vi "仁莫密封检测系统.vi"() -> ()   [LabVIEW 2020]
uses:
  <vilib>/event_ctls.llb/eventvkey.ctl
  <vilib>/NI/Modbus Library/API/Master/Modbus Master.lvclass
  <vilib>/Utility/file.llb/Read Delimited Spreadsheet (string).vi
  <vilib>/NI/Modbus Library/Transmission Data Unit/RTU/RTU Data Unit.lvclass
  <vilib>/NI/Modbus Library/Master Function Definition/Master Function Definition.lvclass
  <vilib>/NI/Modbus Library/Network Protocol/Network Master/Serial/Serial Master.lvclass
panel:
  in  "扫码数据":string
  out "MES状态":bool
  out "通讯状态":bool
  out "刷新按钮":bool
  out "参数组别":string
  out "测试时间":string
  out "实时压力":string
  out "泄露压力":string
  out "门限压力":string
  out "目标压力":string
  out "测试 NG":string
  out "测试 OK":string
  out "测试结果":string
  out "测试总量":string
  out "实时压力(图)":dbl(graph)
  in  "清除计数":bool
  in  "设备启动":bool
  out "消息框":string
  in  "设备停止":bool
  in  "阻断通讯":bool=TRUE
  out "运行状态":string
  out "失败原因":string
  in  "Exit":bool
  # "仁 莫 密 封 检 测 系 统"
  # "S"
  # "Pa"
  # "Pa"
  # "Pa"
  # "Pa"
  # "pcs"
  # "pcs"
  # "pcs"
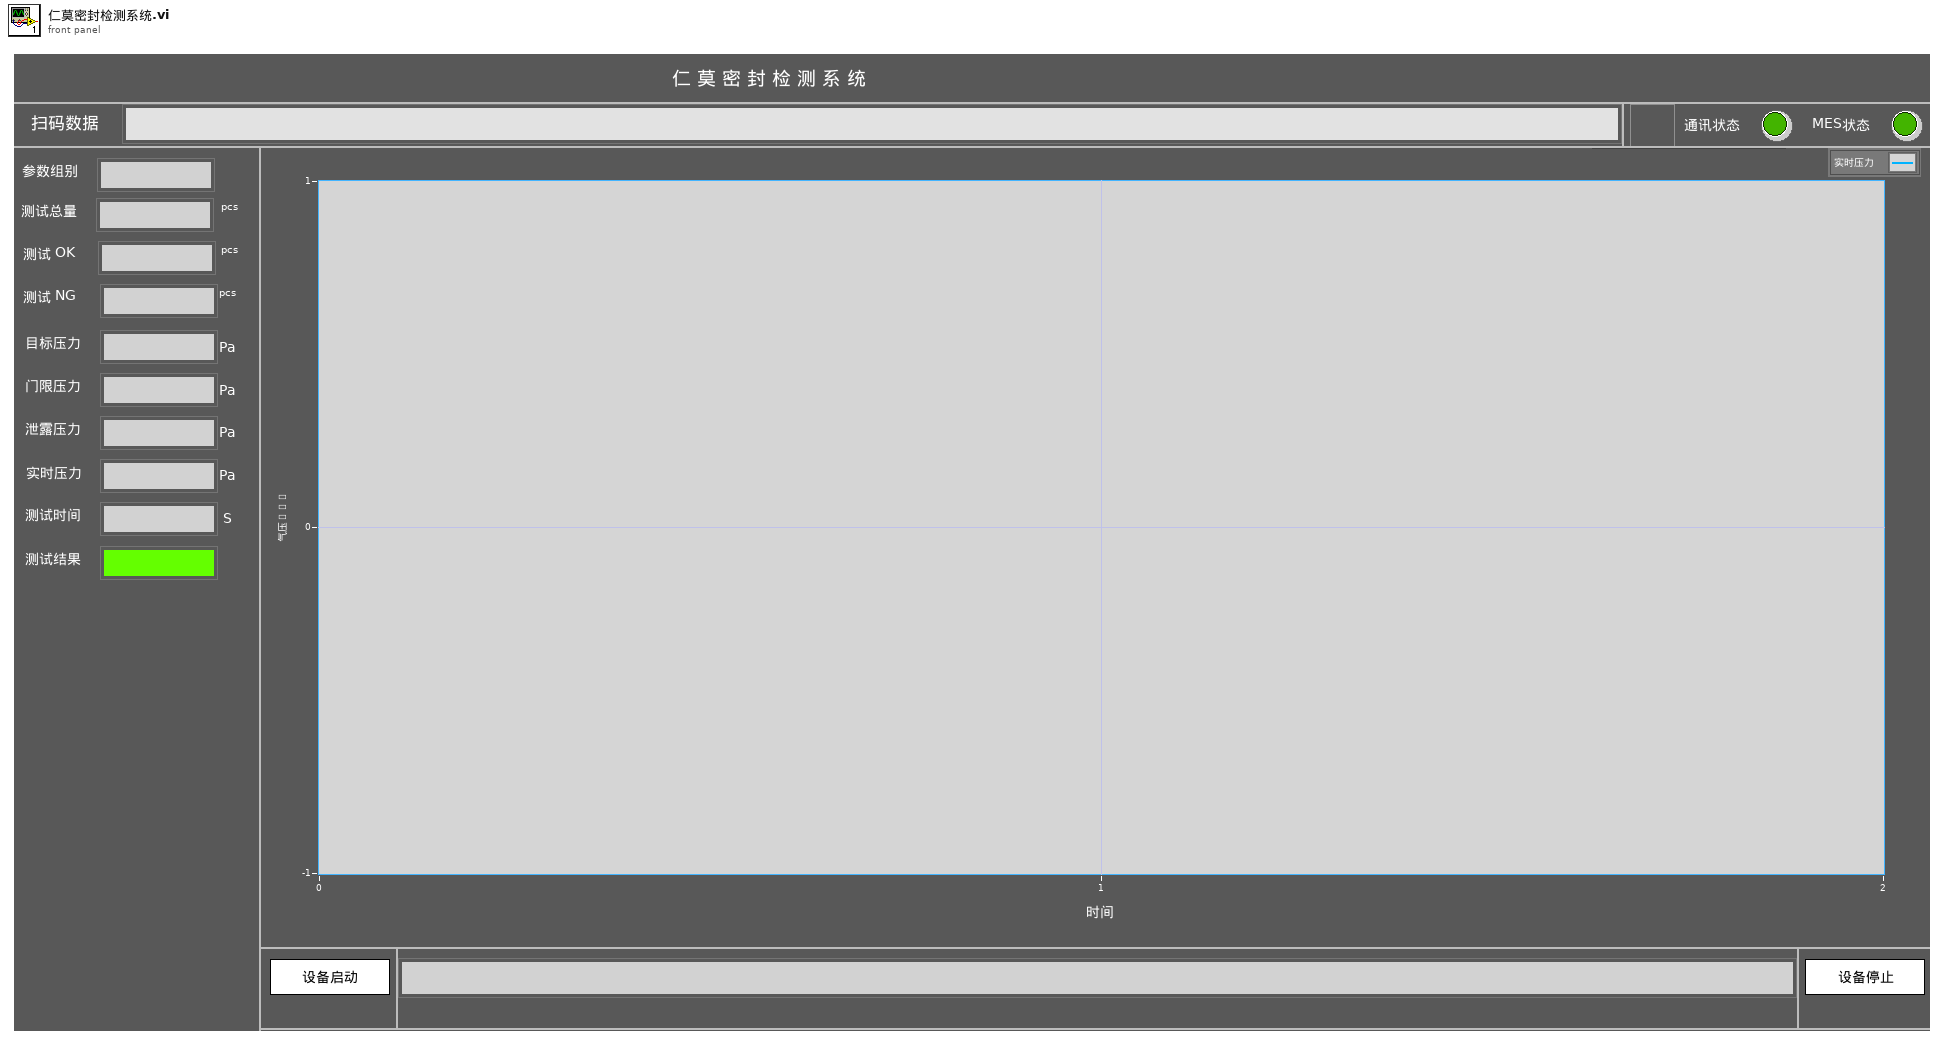
[diagram p1: front panel]
types:
  T1 = typedef "eventvkey.ctl" = enum16{"ASCII", "Enter", "Return", "Shift", "Ctrl", "Alt", "Cmd", "Opt", "Caps", "NumLock", "Clear", "Break", "Up", "Down", "Left", "Right", "Insert", "Delete", "Home", "End", "PageUp", "PageDown", "Escape", "Help", "Pause", "ScrollLock", "F1", "F2", "F3", "F4", "F5", "F6", "F7", "F8", "F9", "F10", "F11", "F12", "F13", "F14", "F15", "F16", "F17", "F18", "F19", "F20", "F21", "F22", "F23", "F24", "Play", "VolumeUp", "VolumeDown", "Mute", "Two Byte Char"}
  T2 = cluster{"地址":u16, "数量":u16, "寄存器值":u16[], "产品总数":string}[]
  T3 = enum32{"Invalid", "Standard", "Closed", "Hidden", "Minimized", "Maximized"}
  T4 = enum32{"invalid app kind", "Development System", "Run Time System", "Student Edition", "Embedded LabVIEW", "Evaluation", "Custom"}
  T5 = cluster{"地址":u16, "数量":u16, "寄存器值":u16[], "名称":string}[]
  T6 = cluster{"读取信息簇":cluster{"地址":u16, "数量":u16, "寄存器值":u16[], "名称":string}, "值解析":string}[]
  T7 = cluster{"温度instance":refnum<class "Modbus Master.lvclass">, "Core":cluster{"Current VI Reference":refnum<vi>, "Close Panel on Exit?":bool}, "serial master instance":refnum<class "Modbus Master.lvclass">, "进站OK":bool, "连接成功":bool, "正在运行":bool, "用户登录":bool, "A读保持寄存器信息组":cluster{"地址":u16, "数量":u16, "寄存器值":u16[], "名称":string}[], "A写入线圈信息组":cluster{"地址":u16, "布尔":bool, "名称":string}[], "A读多组线圈信息组":cluster{"地址":u16, "数量":u16, "名称":string, "线圈组":bool[]}[]}
  T8 = cluster{"连接成功":bool, "MB_实体":refnum<class "Modbus Master.lvclass">}
  T9 = cluster{"地址":u16, "数量":u16, "名称":string, "线圈组":bool[]}[]
  T10 = cluster{"Current VI Reference":refnum<vi>, "Close Panel on Exit?":bool}
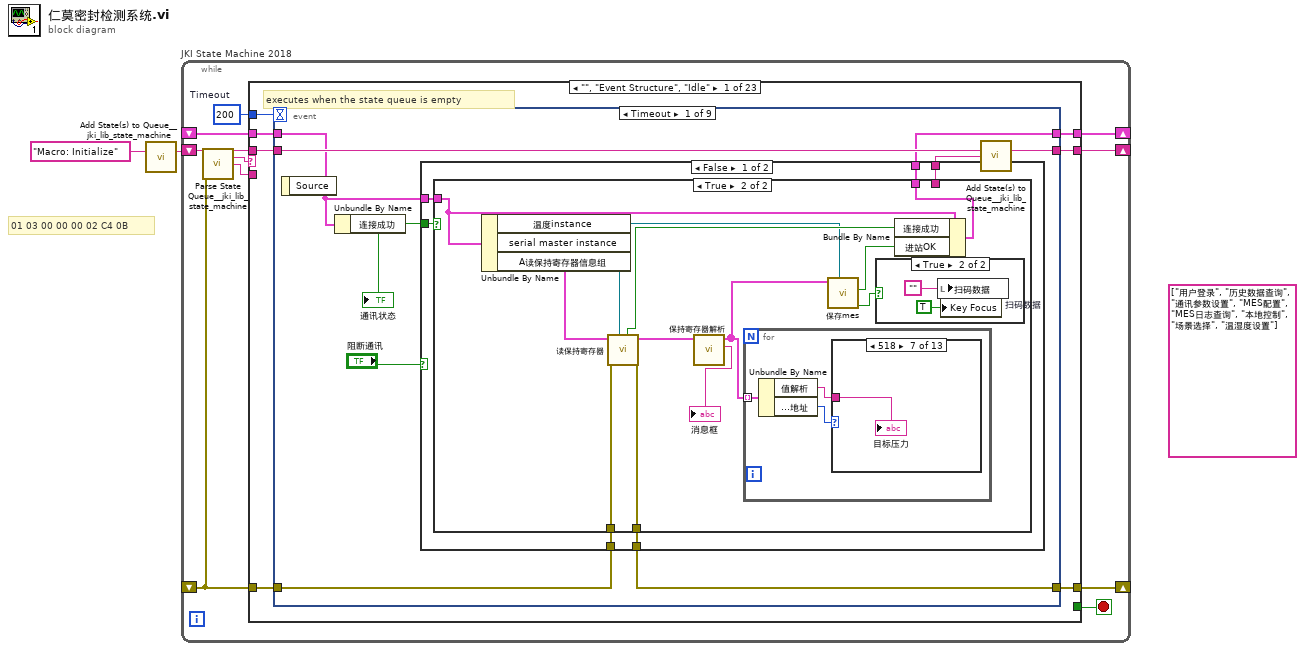
[diagram p0: block diagram]
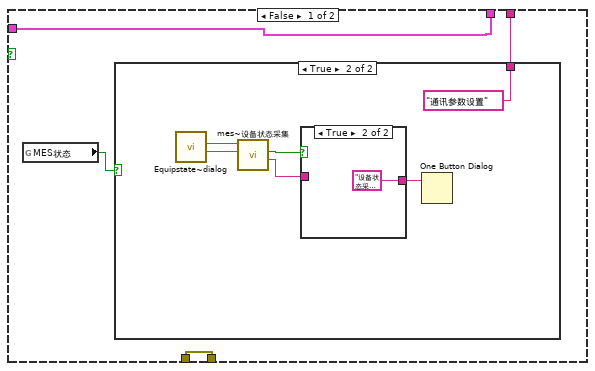
[diagram p2: hidden frame]
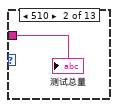
[diagram p7: hidden frame]
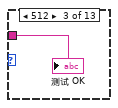
[diagram p8: hidden frame]
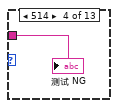
[diagram p9: hidden frame]
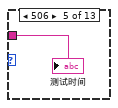
[diagram p10: hidden frame]
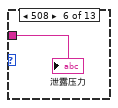
[diagram p11: hidden frame]
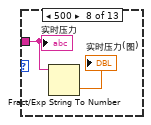
[diagram p12: hidden frame]
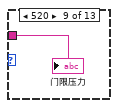
[diagram p13: hidden frame]
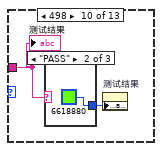
[diagram p14: hidden frame]
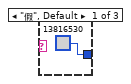
[diagram p15: hidden frame]
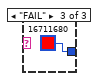
[diagram p16: hidden frame]
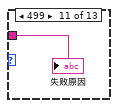
[diagram p17: hidden frame]
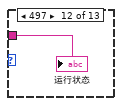
[diagram p18: hidden frame]
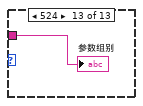
[diagram p19: hidden frame]
diagram:
  (unwired) string[] ["用户登录", "历史数据查询", "通讯参数设置", "MES配置", "MES日志查询", "本地控制", "场景选择", "温湿度设置"] ("L10n_item tags 1")
  # "01 03 00 00 00 02 C4 0B"
  n1 = call <vilib>:"Add State(s) to Queue__jki_lib_state_machine.vi"("State(s) in (\"\")"="Macro: Initialize") -> ("States Out"=w2:string)  [unwired: 14 in]
  n2 = while "JKI State Machine 2018" {
    shift-right: [w6] -> _
    shift-left: _ -> [w5]
    shift-right: [w9] -> _
    shift-left: _ -> [w3]
    shift-right: [w8] -> _
    shift-left: w2 -> [w10]
    stop <- w7 stop-if-true
    w4 = 200  # Timeout
    n3 = call <vilib>:"Parse State Queue__jki_lib_state_machine.vi"("State Queue"=w10, "Error In (no error)"=w3) -> ("Remaining States"=w12:string, "Current State"=w13:string, "Arguments"=w11:string)  [unwired: 11 in]
    n4 = case shown="\"\", \"Event Structure\", \"Idle\"" w13 {
      selector: w13 -> [_ _ w224 _ _ _ _ _ _ _ _ _ _ _ _ _ _ _ _ _ _ _ _]
      tunnel: w12 -> [w20 w223 w228 w247 w254 w259 w263 w284 w292 w296 w310 w316 w327 w396 w401 w411 w416 w432 w458 w507 w550 w562 w567]
      tunnel: w11 -> [_ _ _ _ _ _ _ _ _ _ _ w311 w321 _ _ _ _ _ _ _ _ _ _]
      tunnel: w5 -> [w18 w220 w226 w240 w251 w257 w260 _ w288 w293 w308 w314 w323 w393 w398 w408 w413 w426 w452 w501 w543 w559 w564]
      tunnel: [w17 w221 w230 w244 errorcluster {"status"=FALSE, "code"=0, "source"=""} ("error out") w256 w261 w281 w289 w294 w307 w312 w324 w394 w399 w409 w414 w422 w455 w504 w547 w560 w565] -> w9
      tunnel: w3 -> [w16 w221 w229 w244 w249 w256 w261 w281 w286 w294 w307 w313 w325 w394 w399 w409 w414 w429 w456 w505 w548 w560 w565]
      tunnel: [w19 w222 w227 w246 w253 w258 w262 w283 w291 w295 w309 w315 w326 w395 w400 w410 w415 w431 w457 w506 w549 w561 w566] -> w8
      tunnel: [_ _ _ _ _ TRUE _ _ _ _ _ _ _ _ _ _ _ _ _ _ _ _ _] -> w7
      tunnel: [w15 w220 w226 w245 w251 w257 w260 w282 w288 w293 w308 w314 w323 w393 w398 w408 w413 w424 w450 w499 w544 w559 w563] -> w6
      tunnel: w4 -> [w14 _ _ _ _ _ _ _ _ _ _ _ _ _ _ _ _ _ _ _ _ _ _]
      frame "", "Event Structure", "Idle" {
        # "executes when the state queue is empty"
        n5 = event shown="[0] Timeout" {
          selector: _ -> [_ _ _ _ _ _ _ _ _]
          dyn-events: _ -> [_ _ _ _ _ _ _ _ _]
          timeout: w14 -> [_ _ _ _ _ _ _ _ _]
          tunnel: w20 -> [w29 w89 w94 w100 w181 w193 w203 w213 w219]
          tunnel: [w28 w88 w93 w99 w180 w194 w202 w212 w218] -> w19
          tunnel: w18 -> [w27 w86 w91 w96 w177 w192 w198 w210 w216]
          tunnel: [w25 w87 w92 w98 w179 w191 w195 w211 w217] -> w17
          tunnel: w16 -> [w26 w87 w92 w98 w179 w191 w196 w211 w217]
          tunnel: [w24 w86 w91 w95 w176 w192 w197 w210 w216] -> w15
          event Timeout {
            n6 = event-data() -> ()  [unwired: 1 in, 1 out]
            n7 = Unbundle By Name(w27) -> ("连接成功"=w22:bool)
            "通讯状态" <- w22
            n8 = case shown="False" "阻断通讯" {
              tunnel: w22 -> [w35 _]
              tunnel: w27 -> [w34 w83]
              tunnel: w26 -> [w33 w84]
              tunnel: [w32 w84] -> w25
              tunnel: [w31 w83] -> w24
              tunnel: [w30 _] -> w21
              frame False {
                n9 = case shown="True" w35 {
                  tunnel: w34 -> [w37 w58]
                  tunnel: w33 -> [w39 w60]
                  tunnel: [w39 w59] -> w32
                  tunnel: [w37 w52] -> w31
                  tunnel: [w36 _] -> w30
                  frame False {
                    n10 = global read "Global.vi" "MES状态"() -> (w38:bool)
                    n11 = case shown="True" w38 {
                      tunnel: [_ "通讯参数设置"] -> w36
                      frame False {
                      }
                      frame True {
                        n12 = call "Equipstate~dialog.vi"() -> ("RecordDate"=w44:string, "Equipstate"=w45:string)  [unwired: 10 in]
                        n13 = call "mes~设备状态采集.vi"("RecordDate"=w44, "设备状态"=w45) -> ("ErrorMessage"=w42:string, "设备状态采集成功"=w43:bool)  [unwired: 7 in, 1 out]
                        n14 = case shown="True" w43 {
                          tunnel: w42 -> [w46 _]
                          tunnel: [w46 "设备状态采集成功。"] -> w41
                          frame False {
                          }
                          frame True {
                          }
                        }
                        n15 = One Button Dialog(message=w41) -> ()  [unwired: 1 in, 1 out]
                      }
                    }
                  }
                  frame True {
                    n16 = Unbundle By Name(w58) -> ("温度instance"=w49:refnum<class "Modbus Master.lvclass">, "serial master instance"=w57:refnum<class "Modbus Master.lvclass">, "A读保持寄存器信息组"=w56:T5)
                    n17 = call "读保持寄存器.vi"("MB_实体"=w57, "error in"=w60, "读保持寄存器信息组__输入"=w56) -> ("输出簇"=w59:errorcluster, "读保持寄存器信息组_输出"=w54:T5, "连接成功"=w55:bool)  [unwired: 6 in]
                    n18 = call "保持寄存器解析.vi"("A读保持寄存器信息组"=w54) -> ("运行状态"=→"消息框":string, "参数值"=w51:T6)  [unwired: 9 in]
                    n19 = for {
                      tunnel: w51 -> [w64] mode=indexing
                      n20 = Unbundle By Name(w64) -> ("值解析"=w63:string, "读取信息簇.地址"=w65:u16)
                      n21 = case shown="518" w65 {
                        tunnel: w63 -> [_ w66 w67 w68 w69 w70 w71 w73 w74 w76 w80 w81 w82]
                        frame Default {
                        }
                        frame 510 {
                          "测试总量" <- w66
                        }
                        frame 512 {
                          "测试 OK" <- w67
                        }
                        frame 514 {
                          "测试 NG" <- w68
                        }
                        frame 506 {
                          "测试时间" <- w69
                        }
                        frame 508 {
                          "泄露压力" <- w70
                        }
                        frame 518 {
                          "目标压力" <- w71
                        }
                        frame 500 {
                          n22 = Fract/Exp String To Number(string=w73) -> (number=→"实时压力(图)":dbl)  [unwired: 3 in, 1 out]
                          "实时压力" <- w73
                        }
                        frame 520 {
                          "门限压力" <- w74
                        }
                        frame 498 {
                          n23 = case shown="\"PASS\"" w76 {
                            tunnel: [u32 13816530 ("颜色盒") u32 6618880 u32 16711680] -> w75
                            frame "假", Default {
                            }
                            frame "PASS" {
                            }
                            frame "FAIL" {
                            }
                          }
                          n24 = property on="测试结果" class="Str"("Text.BGColor"=w75) -> ()  [unwired: 2 in, 2 out]
                          "测试结果" <- w76
                        }
                        frame 499 {
                          "失败原因" <- w80
                        }
                        frame 497 {
                          "运行状态" <- w81
                        }
                        frame 524 {
                          "参数组别" <- w82
                        }
                      }
                    }
                    n25 = call "保存mes.vi"("温度instance"=w49, "参数值"=w51) -> ("已保存?"=w48:bool, "进站OK?"=w50:bool)  [unwired: 8 in]
                    n26 = case shown="True" w48 {
                      frame False {
                      }
                      frame True {
                        n27 = local write "扫码数据"("") -> ()
                        n28 = property on="扫码数据" class="Str"("Key Focus"=TRUE) -> ()  [unwired: 2 in, 2 out]
                      }
                    }
                    n29 = Bundle By Name(cluster=w58, "连接成功"=w55, "进站OK"=w50) -> (w52:T7)
                  }
                }
              }
              frame True {
              }
            }
            n30 = call <vilib>:"Add State(s) to Queue__jki_lib_state_machine.vi"("State(s) in (\"\")"=w29, "State(s) at Back (\"\")"=w21) -> ("States Out"=w28:string)  [unwired: 13 in]
          }
          event "设备启动": Value Change {
            n31 = event-data() -> ()  [unwired: 1 in, 1 out]
            n32 = call <vilib>:"Add State(s) to Queue__jki_lib_state_machine.vi"("State(s) in Front (\"\")"="//Communication: 读运行标志\nCommunication: 设备启动\n//Communication: 读运行标志", "State(s) in (\"\")"=w89) -> ("States Out"=w88:string)  [unwired: 13 in]
          }
          event "设备停止": Value Change {
            n33 = event-data() -> ()  [unwired: 1 in, 1 out]
            n34 = call <vilib>:"Add State(s) to Queue__jki_lib_state_machine.vi"("State(s) in Front (\"\")"="//Communication: 读运行标志\nCommunication: 设备停止\n//Communication: 读运行标志", "State(s) in (\"\")"=w94) -> ("States Out"=w93:string)  [unwired: 13 in]
          }
          event Menu Selection (User) {
            n35 = event-data() -> ("ItemTag"=w97:string)  [unwired: 1 in]
            n36 = case shown="\"本地控制\"" w97 {
              tunnel: w96 -> [w101 w104 w112 w123 w135 w137 w148 w161 w166]
              tunnel: [w101 w103 w112 w123 w135 w136 w147 w161 w165] -> w95
              frame "假", Default {
              }
              frame "用户登录" {
                n37 = call "mes~Login Dialog.vi"() -> ("Success?"=w102:bool)  [unwired: 10 in, 1 out]
                n38 = Bundle By Name(cluster=w104, "用户登录"=w102) -> (w103:T7)
                n39 = case shown="True" w102 {
                  frame False {
                    n40 = Current VI's Menubar() -> (w106:refnum<k9>)
                    n41 = Delete Menu Items(9:w106) -> (3:w105:refnum<k9>)  [unwired: 3 in, 1 out]
                    n42 = Insert Menu Items(7:string[] ["用户登录", "历史数据查询", "MES配置", "MES日志查询", "本地控制", "温湿度设置"] ("L10n_item tags 1"), 9:w105) -> ()  [unwired: 4 in, 3 out]
                  }
                  frame True {
                    n43 = Current VI's Menubar() -> (w110:refnum<k9>)
                    n44 = Delete Menu Items(9:w110) -> (0:w108:errorcluster, 3:w109:refnum<k9>)  [unwired: 3 in]
                    n45 = Insert Menu Items(6:w108, 7:string[] ["用户登录", "历史数据查询", "通讯参数设置", "MES配置", "MES日志查询", "本地控制"] ("L10n_item tags 1"), 9:w109) -> ()  [unwired: 3 in, 3 out]
                  }
                }
              }
              frame "历史数据查询" {
                n46 = stacked-sequence {
                  frame #0 {
                    n47 = call <vilib>:"Check if File or Folder Exists.vi"("path"=path "D:/MES" ("路径")) -> ("file or folder exists?"=w115:bool, "dup path"=w114:path)  [unwired: 8 in, 1 out]
                    n48 = case shown="False" w115 {
                      tunnel: w114 -> [w117 w118]
                      tunnel: [w116 w118] -> _
                      frame False {
                        n49 = Create Folder(path (use dialog)=w117) -> (created path=w116:path)  [unwired: 2 in, 2 out]
                      }
                      frame True {
                      }
                    }
                  }
                  frame #1 {
                    n50 = call <vilib>:"Space Constant.vi"() -> ("String"=w120:string)
                    n51 = Concatenate Strings("explorer" ("字符串"), w120, "D:\\MES" ("字符串")) -> (w122:string)
                    n52 = call <vilib>:"System Exec.vi"("command line"=w122) -> ()  [unwired: 7 in, 4 out]
                  }
                }
              }
              frame "MES日志查询" {
                n53 = stacked-sequence {
                  frame #0 {
                    n54 = call <vilib>:"Check if File or Folder Exists.vi"("path"=path "D:/Log" ("路径")) -> ("file or folder exists?"=w126:bool, "dup path"=w125:path)  [unwired: 8 in, 1 out]
                    n55 = case shown="False" w126 {
                      tunnel: w125 -> [w128 w129]
                      tunnel: [w127 w129] -> _
                      frame False {
                        n56 = Create Folder(path (use dialog)=w128) -> (created path=w127:path)  [unwired: 2 in, 2 out]
                      }
                      frame True {
                      }
                    }
                  }
                  frame #1 {
                    n57 = call <vilib>:"Space Constant.vi"() -> ("String"=w131:string)
                    n58 = Concatenate Strings("explorer" ("字符串"), w131, "D:\\Log" ("字符串")) -> (w133:string)
                    n59 = call <vilib>:"System Exec.vi"("command line"=w133) -> ()  [unwired: 7 in, 4 out]
                  }
                }
              }
              frame "MES配置" {
                n60 = call "mes配置前验证.vi"() -> ("Success?"=w134:bool)  [unwired: 10 in, 1 out]
                n61 = case shown="True" w134 {
                  frame False {
                  }
                  frame True {
                    n62 = call "mes参数配置.vi"() -> ()  [unwired: 11 in, 1 out]
                  }
                }
              }
              frame "通讯参数设置" {
                n63 = stacked-sequence {
                  tunnel: w137 -> [_ w142 _]
                  tunnel: [_ w139 _] -> w136
                  frame #0 {
                    n64 = local write "阻断通讯"(TRUE ("阻断通讯")) -> ()
                  }
                  frame #1 {
                    n65 = call "通讯参数设置.vi"() -> ("A设备簇"=w143:T8)  [unwired: 5 in]
                    n66 = Unbundle By Name(w143) -> ("MB_实体"=w141:refnum<class "Modbus Master.lvclass">, "连接成功"=w140:bool)
                    n67 = Bundle By Name(cluster=w142, "serial master instance"=w141, "连接成功"=w140) -> (w139:T7)
                  }
                  frame #2 {
                    n68 = local write "阻断通讯"(FALSE ("阻断通讯")) -> ()
                  }
                }
              }
              frame "本地控制" {
                n69 = call "本地控制.vi"() -> ("远程2"=w146:bool)  [unwired: 11 in]
                "MES状态" <- w146
                n70 = Not(x=w146) -> (.not. x?=w145:bool)
                n71 = Bundle By Name(cluster=w148, "用户登录"=w145, "进站OK"=w145) -> (w147:T7)
                n72 = global write "Global.vi" "MES状态"(w146) -> ()
                n73 = global write "Global.vi" "产品进站"(w145) -> ()
                n74 = case shown="True" w146 {
                  frame False {
                    n75 = Current VI's Menubar() -> (w150:refnum<k9>)
                    n76 = Delete Menu Items(9:w150) -> (3:w149:refnum<k9>)  [unwired: 3 in, 1 out]
                    n77 = Insert Menu Items(7:string[] ["历史数据查询", "通讯参数设置", "MES配置", "MES日志查询", "本地控制"] ("L10n_item tags 1"), 9:w149) -> ()  [unwired: 4 in, 3 out]
                  }
                  frame True {
                    n78 = Current VI's Menubar() -> (w154:refnum<k9>)
                    n79 = Delete Menu Items(9:w154) -> (0:w152:errorcluster, 3:w153:refnum<k9>)  [unwired: 3 in]
                    n80 = Insert Menu Items(6:w152, 7:string[] ["用户登录", "历史数据查询", "通讯参数设置", "MES配置", "MES日志查询", "本地控制"] ("L10n_item tags 1"), 9:w153) -> ()  [unwired: 3 in, 3 out]
                  }
                }
              }
              frame "场景选择" {
                n81 = call "Equipstate~dialog.vi"() -> ("RecordDate"=w159:string, "Equipstate"=w160:string)  [unwired: 10 in]
                n82 = call "mes~设备状态采集.vi"("RecordDate"=w159, "设备状态"=w160) -> ("ErrorMessage"=w157:string, "设备状态采集成功"=w158:bool)  [unwired: 7 in, 1 out]
                n83 = case shown="True" w158 {
                  tunnel: w157 -> [w162 _]
                  tunnel: [w162 "设备状态采集正常。"] -> w156
                  frame False {
                  }
                  frame True {
                  }
                }
                n84 = One Button Dialog(message=w156) -> ()  [unwired: 1 in, 1 out]
              }
              frame "温湿度设置" {
                n85 = call "通讯参数设置.vi"("波特率"=u32 9600) -> ("A设备簇"=w168:T8)  [unwired: 4 in]
                n86 = Unbundle By Name(w168) -> ("MB_实体"=w167:refnum<class "Modbus Master.lvclass">)
                n87 = Bundle By Name(cluster=w166, "温度instance"=w167) -> (w165:T7)
              }
            }
            n88 = call <vilib>:"Add State(s) to Queue__jki_lib_state_machine.vi"("State(s) in (\"\")"=w100) -> ("States Out"=w99:string)  [unwired: 14 in]
          }
          event "扫码数据": Key Down {
            n89 = event-data() -> ("VKey"=w175:T1)  [unwired: 1 in]
            n90 = Equal?(x=w175, y=eventvkey."Return" ("V键")) -> (x = y?=w173:bool)
            n91 = case shown="True" w173 {
              tunnel: [FALSE ("进站成功") w183] -> w172
              frame False {
              }
              frame True {
                n92 = global read "Global.vi" "MES状态"() -> (w184:bool)
                n93 = case shown="False" w184 {
                  tunnel: "扫码数据" -> [_ w189]
                  tunnel: [TRUE ("进站成功") w188] -> w183
                  frame False {
                  }
                  frame True {
                    n94 = call "mes~产品进站.vi"("identification"=w189) -> ("ErrorMessage"=w187:string, "进站成功"=w188:bool)  [unwired: 8 in, 1 out]
                    n95 = case shown="True" w188 {
                      tunnel: w187 -> [_ _]
                      frame False {
                        n96 = One Button Dialog(message="产品进站失败。") -> ()  [unwired: 1 in, 1 out]
                      }
                      frame True {
                        (unwired) "产品进站成功。"
                      }
                    }
                  }
                }
                n97 = global write "Global.vi" "PACK编码"("扫码数据") -> ()
              }
            }
            n98 = global write "Global.vi" "产品进站"(w172) -> ()
            n99 = Bundle By Name(cluster=w177, "进站OK"=w172) -> (w176:T7)
            n100 = Select(t="Communication: 设备启动", s=w172, f="") -> (s? t:f=w170:string)
            n101 = call <vilib>:"Add State(s) to Queue__jki_lib_state_machine.vi"("State(s) in (\"\")"=w181, "State(s) at Back (\"\")"=w170) -> ("States Out"=w180:string)  [unwired: 13 in]
            "刷新按钮" <- FALSE ("刷新按钮")
          }
          event "扫码数据": Mouse Down {
            n102 = event-data() -> ()  [unwired: 1 in, 1 out]
            n103 = call <vilib>:"Add State(s) to Queue__jki_lib_state_machine.vi"("State(s) in (\"\")"=w193) -> ("States Out"=w194:string)  [unwired: 14 in]
          }
          event "清除计数": Value Change {
            n104 = event-data() -> ()  [unwired: 1 in, 1 out]
            n105 = local write "清除计数"(FALSE) -> ()
            n106 = Unbundle By Name(w198) -> ("serial master instance"=w199:refnum<class "Modbus Master.lvclass">)
            n107 = disable-structure shown="Disabled" {
              disable-tunnel: [w208 _] -> w200
              disable-tunnel: w199 -> [w207 _]
              disable-tunnel: w196 -> [w205 _]
              disable-tunnel: [w204 _] -> w195
              frame Disabled {
                n108 = call "写保持寄存器.vi"("MB_实体"=w207, "error in"=w205, "读保持寄存器信息组__输入"=T2 [{"地址"=510, "数量"=2, "寄存器值"=[0, 0], "产品总数"="产品总数"}, {"地址"=512, "数量"=2, "寄存器值"=[0, 0], "产品总数"="合格数量"}, {"地址"=514, "数量"=2, "寄存器值"=[0, 0], "产品总数"="泄露数量"}]) -> ("输出簇"=w204:errorcluster, "连接成功"=w208:bool)  [unwired: 7 in]
              }
              frame Enabled {
              }
            }
            n109 = Bundle By Name(cluster=w198, "连接成功"=w200) -> (w197:T7)
            n110 = call <vilib>:"Add State(s) to Queue__jki_lib_state_machine.vi"("State(s) in (\"\")"=w203) -> ("States Out"=w202:string)  [unwired: 14 in]
          }
          event "Exit": Value Change {
            # "Exit Button Value Change (pressed) Event\n(this executes Macro: Exit to terminate the VI)"
            n111 = event-data() -> ()  [unwired: 1 in, 1 out]
            n112 = call <vilib>:"Add State(s) to Queue__jki_lib_state_machine.vi"("State(s) in Front (\"\")"="Macro: Exit", "State(s) in (\"\")"=w213) -> ("States Out"=w212:string)  [unwired: 13 in]
          }
          event Panel Close? {
            # "Discard the event because we'll close the front panel ourselves in Macro: Exit"
            # "Close Panel button (pressed) Event\n(this executes Macro: Exit to terminate the VI)"
            n113 = event-data() -> ()  [unwired: 1 in, 1 out]
            n114 = event-data("Discard?"=TRUE) -> ()  [unwired: 1 in, 1 out]
            n115 = call <vilib>:"Add State(s) to Queue__jki_lib_state_machine.vi"("State(s) in Front (\"\")"="Macro: Exit", "State(s) in (\"\")"=w219) -> ("States Out"=w218:string)  [unwired: 13 in]
          }
        }
      }
      frame "---------- Core ----------" {
        # "Do not put any code in this frame.\n(it is a separator no-op)"
        n116 = call <vilib>:"Add State(s) to Queue__jki_lib_state_machine.vi"("State(s) in (\"\")"=w223) -> ("States Out"=w222:string)  [unwired: 14 in]
      }
      frame Default {
        w233 = 42 items=["No error", "Argument error", "Memory is full", "Out of zone", "End of file", "File already open", "Generic file I/O error", "File not found", "File permission error", "Disk is full", "Duplicate path", "Too many files open", "System feature not enabled", "Resource file not found", "Cannot add resource", "Resource not found", "Image not found", "Image memory error", "Pen does not exist", "Config type invalid", "Config token not found", "Config parse error", "Config memory error", "Bad external code format", "Bad external code offset", "External code not present", "Null window", "Destroy window error", "Null menu", "Print aborted", "Bad print record", "Print driver error", "Windows error during printing", "Memory error during printing", "Print dialog error", "Generic print error", "Invalid device refnum", "Device not found", "Device parameter error", "Device unit error", "Cannot open device", "Device call aborted", "Generic error", "Cancelled by user", "Object ID too low", "Object ID too high", "Object not in heap", "Unknown heap", "Unknown object (invalid DefProc)", "Unknown object (DefProc not in table)", "Message out of range", "Invalid (null) method", "Unknown message", "Manager call not supported", "Bad address", "Network operation in progress", "Network operation timed out", "Connection is busy", "Network attribute not supported", "Network error", "Address in use", "System out of memory", "Connection aborted", "Connection refused", "Not connected", "Already connected", "Connection closed", "Initialization error (interapplication manager)", "Bad occurrence", "Wait on unbound occurrence handler", "Occurrence queue overflow", "Datalog type conflict", "Unused", "Unrecognized type (interapplication manager)", "Memory corrupt", "Failed to make temporary DLL", "Old CIN version", "Drag socket not found", "Failed to load drop-object", "Failed to register OLE object", "Failed to release OLE object", "Format specifier type mismatch", "Unknown format specifier", "Too few format specifiers", "Too many format specifiers", "Scan failed", "Newer CIN version", "Error converting to variant", "Runtime menu error", "Password tampered", "Variant attribute not found", "Incompatible variant data type", "Event data is not available", "Event Store is not present", "Occurrence is not found", "Event Queue is not created", "Event info is not available", "Refnum passed is NULL", "Error retrieving Class GUID", "Error retrieving CoClass GUID", "Error retrieving TypeLib GUID.", "Bad built application magic bytes.", "Specific driver is different from the specific driver associated with the Logical Name.", "There is no session opened to the class driver.", "Max Error", "MAX - Error with config objects", "MAX - Error loading configuration", "MAX - Group not supported"]
        # "Current State"
        # "Do not delete, rename, or modify this frame.\n(this is used to capture unhandled states and typos)"
        # "Handle mistyped state name (developer tool)"
        n117 = Format Into String(format string="Software Exception: Unhandled State \"%s\"." ("message"), error in=w229, w224) -> (resulting string=w232:string, error out=w231:errorcluster)  [unwired: 1 in]
        n118 = call <vilib>:"Error Cluster From Error Code.vi"("show call chain? (False)"=TRUE, "error in (no error)"=w231, "error message (\"\")"=w232, "error code (0)"=w233) -> ("error out"=w230:errorcluster)  [unwired: 5 in]
        n119 = call <vilib>:"Add State(s) to Queue__jki_lib_state_machine.vi"("State(s) in (\"\")"=w228) -> ("States Out"=w227:string)  [unwired: 14 in]
      }
      frame "Initialize Core Data" {
        # "Do not delete, rename, or modify this frame.\n(this is used to determine panel behavior on exit)"
        # "originally closed?"
        # "exe?"
        # "If panel starts closed or is an EXE, then close it when we exit"
        n120 = property class="VI"() -> ("FP.State"=w237:T3)  [unwired: 2 in, 2 out]
        n121 = property class="App"() -> ("App.Kind"=w243:T4)  [unwired: 2 in, 2 out]
        n122 = control-ref of="Current VI Reference"() -> (w238:refnum<vi>)
        n123 = Equal?(x=w237, y=T3."Closed" ("Front Panel Window:State")) -> (x = y?=w235:bool)
        n124 = Equal?(x=w243, y=T4."Run Time System" ("Application:Kind")) -> (x = y?=w241:bool)
        n125 = Or(x=w235, y=w241) -> (x .or. y?=w239:bool)
        n126 = Bundle By Name(cluster=w240, "Core.Current VI Reference"=w238, "Core.Close Panel on Exit?"=w239) -> (w245:T7)
        n127 = call <vilib>:"Add State(s) to Queue__jki_lib_state_machine.vi"("State(s) in (\"\")"=w247) -> ("States Out"=w246:string)  [unwired: 14 in]
      }
      frame "Error Handler" {
        # "Handle any errors here.\nYou can also output any states to clean-up after errors occur"
        # "Clear error"
        n128 = Unbundle By Name(w249) -> ("source"=w248:string)
        n129 = One Button Dialog(message=w248) -> ()  [unwired: 1 in, 1 out]
        n130 = call <vilib>:"Add State(s) to Queue__jki_lib_state_machine.vi"("State(s) in Front (\"\")"="/* Post Error States", "State(s) in (\"\")"=w254) -> ("States Out"=w253:string)  [unwired: 13 in]
      }
      frame "Exit" {
        # "Do not put any code in this frame.\n(No errors that occur here will be handled.)"
        n131 = call <vilib>:"Add State(s) to Queue__jki_lib_state_machine.vi"("State(s) in (\"\")"=w259) -> ("States Out"=w258:string)  [unwired: 14 in]
      }
      frame "---------- Data ----------" {
        # "Do not put any code in this frame.\n(It is a separator no-op. You can make a copy of this frame to create a new Data frame)"
        n132 = call <vilib>:"Add State(s) to Queue__jki_lib_state_machine.vi"("State(s) in (\"\")"=w263) -> ("States Out"=w262:string)  [unwired: 14 in]
      }
      frame "Data: Initialize" {
        w264 = refnum<class "Modbus Master.lvclass"> refnum  # 温度instance
        w265 = FALSE ("MES状态")
        w266 = FALSE  # 进站OK
        w273 = TRUE  # 用户登录
        w274 = FALSE  # 正在运行
        w275 = T5 [{"地址"=510, "数量"=2, "寄存器值"=[0, 0], "名称"="产品总数"}, {"地址"=512, "数量"=2, "寄存器值"=[0, 0], "名称"="合格数量"}, {"地址"=514, "数量"=2, "寄存器值"=[0, 0], "名称"="泄露数量"}, {"地址"=506, "数量"=2, "寄存器值"=[0, 0], "名称"="1测试时间"}, {"地址"=508, "数量"=2, "寄存器值"=[0, 0], "名称"="1测试泄漏"}, {"地址"=518, "数量"=2, "寄存器值"=[0, 0], "名称"="1#目标压力"}, {"地址"=498, "数量"=1, "寄存器值"=[0, 0], "名称"="1#测试结果"}, {"地址"=500, "数量"=2, "寄存器值"=[0, 0], "名称"="实时压力"}, {"地址"=520, "数量"=2, "寄存器值"=[], "名称"="门限压力"}, {"地址"=499, "数量"=1, "寄存器值"=[], "名称"="失败原因"}, {"地址"=497, "数量"=1, "寄存器值"=[], "名称"="运行状态"}, {"地址"=524, "数量"=2, "寄存器值"=[], "名称"="参数组别"}]  # A读保持寄存器信息组
        w276 = T9 [{"地址"=507, "数量"=1, "名称"="1测试结束标志", "线圈组"=[FALSE, TRUE]}]  # A读多组线圈信息组
        w277 = cluster{"地址":u16, "布尔":bool, "名称":string}[] [{"地址"=50, "布尔"=FALSE, "名称"="启动"}, {"地址"=51, "布尔"=FALSE, "名称"="停止"}]  # A写入线圈信息组
        w278 = FALSE  # 连接成功
        w279 = refnum<class "Modbus Master.lvclass"> refnum  # serial master instance
        w280 = T10 {"Current VI Reference"=refnum, "Close Panel on Exit?"=FALSE}  # Core
        # "Initialize the shift-register data, here.\n(data names are defined by what you wire into the bundle function)"
        n133 = call <vilib>:"Application Directory.vi"() -> ("Application Directory"=w271:path)
        n134 = Build Path(base path=w271, name or relative path=path "data/mes.cfg") -> (appended path=w272:path)
        n135 = call-poly <vilib>:"Read Delimited Spreadsheet.vi"("file path (dialog if empty)"=w272, "delimiter (\\t)"="::" ("delimiter (\\t)")) -> ("all rows"=w267:string[][])  [unwired: 8 in, 5 out]
        n136 = call "mes初始化.vi"("mes"=w267) -> ()  [unwired: 11 in]
        n137 = global write "Global.vi" "MES状态"(w265) -> ()
        n138 = global write "Global.vi" "正在运行"(w265) -> ()
        n139 = local write "MES状态"(w265) -> ()
        n140 = global write "Global.vi" "产品进站"(w265) -> ()
        n141 = global write "Global.vi" "运行状态时间点"(dbl[] [0.0, 0.0, 0.0, 0.0, 0.0, 0.0, 0.0, 0.0, 0.0] ("运行状态时间点")) -> ()
        n142 = Bundle("温度instance"=w264, "Core"=w280, "serial master instance"=w279, "进站OK"=w266, "连接成功"=w278, "正在运行"=w274, "用户登录"=w273, "A读保持寄存器信息组"=w275, "A写入线圈信息组"=w277, "A读多组线圈信息组"=w276) -> (w282:T7)  [unwired: 1 in]
        n143 = call <vilib>:"Add State(s) to Queue__jki_lib_state_machine.vi"("State(s) in (\"\")"=w284) -> ("States Out"=w283:string)  [unwired: 14 in]
      }
      frame "Data: Cleanup" {
        # "Cleanup any data and references, here.\n(this is called automatically, by the Macro: Exit)"
        n144 = Unbundle By Name(w288) -> ("Core.Current VI Reference"=w290:refnum<vi>, "serial master instance"=w287:refnum<class "Modbus Master.lvclass">)
        n145 = call-dynamic "Shutdown.vi"("error in"=w286, "Modbus master in"=w287) -> ("error out"=w285:errorcluster)  [unwired: 9 in]
        n146 = Close Reference(reference=w290, error in (no error)=w285) -> (error out=w289:errorcluster)
        n147 = call <vilib>:"Add State(s) to Queue__jki_lib_state_machine.vi"("State(s) in (\"\")"=w292) -> ("States Out"=w291:string)  [unwired: 14 in]
      }
      frame "---------- UI ----------" {
        # "Do not put any code in this frame.\n(It is a separator no-op. You can make a copy of this frame to create a new UI frame)"
        n148 = call <vilib>:"Add State(s) to Queue__jki_lib_state_machine.vi"("State(s) in (\"\")"=w296) -> ("States Out"=w295:string)  [unwired: 14 in]
      }
      frame "UI: Initialize" {
        w303 = ""
        # "Initialize the User Interface, here.\n(this is called automatically, by the Macro: Init)"
        n149 = call "读取配置文件.vi"("配置"="程序名") -> ("error out"=w302:errorcluster, "路径"=w301:string)  [unwired: 9 in]
        n150 = property class="VI"(error in=w302, "Front Panel.Title"=w301) -> (error out=w299:errorcluster)  [unwired: 1 in, 1 out]
        n151 = Current VI's Menubar() -> (w306:refnum<k9>)
        n152 = Delete Menu Items(6:w299, 9:w306) -> (0:w305:errorcluster, 3:w304:refnum<k9>)  [unwired: 2 in]
        n153 = local write "扫码数据"(w303) -> ()
        n154 = global write "Global.vi" "PACK编码"(w303) -> ()
        n155 = Insert Menu Items(6:w305, 7:string[] ["历史数据查询", "通讯参数设置", "MES配置", "MES日志查询", "本地控制"] ("L10n_item tags 1"), 9:w304) -> ()  [unwired: 3 in, 3 out]
        n156 = property on="测试结果" class="Str"("Text.BGColor"=u32 13816530 ("颜色盒")) -> ()  [unwired: 2 in, 2 out]
        n157 = call <vilib>:"Add State(s) to Queue__jki_lib_state_machine.vi"("State(s) in (\"\")"=w310) -> ("States Out"=w309:string)  [unwired: 14 in]
      }
      frame "UI: Cursor Set" {
        # "Argument"
        # "Set and Unset Cursor Busy.\n(Usage: \"UI: Cursor Set >> Busy|Idle\")"
        n158 = case shown="\"Idle\", Default" w311 {
          tunnel: w313 -> [w318 w320]
          tunnel: [w317 w319] -> w312
          frame "Idle", Default {
            n159 = call <vilib>:"Unset Busy.vi"("error in (no error)"=w318) -> ("error out"=w317:errorcluster)  [unwired: 10 in]
          }
          frame "Busy" {
            n160 = call <vilib>:"Set Busy.vi"("error in (no error)"=w320) -> ("error out"=w319:errorcluster)  [unwired: 9 in, 1 out]
          }
        }
        n161 = call <vilib>:"Add State(s) to Queue__jki_lib_state_machine.vi"("State(s) in (\"\")"=w316) -> ("States Out"=w315:string)  [unwired: 14 in]
      }
      frame "UI: Front Panel State" {
        # "Argument"
        # "Set Front Panel Open or Closed\n(Usage: \"UI: Front Panel State >> Open|Close\")"
        n162 = Unbundle By Name(w323) -> ("Core.Current VI Reference"=w322:refnum<vi>)
        n163 = case shown="\"Maximize\", \"Maximized\"" w321 {
          tunnel: w325 -> [w333 w348 w359 w372 w385]
          tunnel: [w335 w349 w361 w374 w387] -> w324
          tunnel: w322 -> [w334 w346 w360 w373 w386]
          frame "Open", "Standard", Default {
            w328 = T3."Standard" ("State")
            n164 = property class="VI"(reference=w334, error in=w333) -> (reference out=w331:refnum<vi>, error out=w332:errorcluster, "FP.State"=w330:T3)
            n165 = Not Equal?(x=w330, y=w328) -> (x != y?=w329:bool)
            n166 = case shown="True" w329 {
              tunnel: [w339 w341] -> w335
              tunnel: w332 -> [w338 w341]
              tunnel: w331 -> [w337 _]
              tunnel: w328 -> [w336 _]
              frame True {
                n167 = invoke class="VI" method="FP.Open"(reference=w337, error in=w338, "Activate"=TRUE, "State"=w336) -> (error out=w339:errorcluster)  [unwired: 1 in, 4 out]
              }
              frame False {
              }
            }
          }
          frame "Close", "Closed" {
            n168 = property class="VI"(reference=w346, error in=w348) -> (reference out=w345:refnum<vi>, error out=w347:errorcluster, "FP.State"=w343:T3)
            n169 = Not Equal?(x=w343, y=T3."Closed" ("Front Panel Window:State")) -> (x != y?=w342:bool)
            n170 = case shown="True" w342 {
              tunnel: [w350 w353] -> w349
              tunnel: w347 -> [w350 w352]
              tunnel: w345 -> [_ w351]
              frame False {
              }
              frame True {
                n171 = invoke class="VI" method="FP.Close"(reference=w351, error in=w352) -> (error out=w353:errorcluster)  [unwired: 1 in, 2 out]
              }
            }
          }
          frame "Hidden", "Hide" {
            w354 = T3."Hidden" ("State")
            n172 = property class="VI"(reference=w360, error in=w359) -> (reference out=w357:refnum<vi>, error out=w358:errorcluster, "FP.State"=w356:T3)
            n173 = Not Equal?(x=w356, y=w354) -> (x != y?=w355:bool)
            n174 = case shown="True" w355 {
              tunnel: [w365 w366] -> w361
              tunnel: w358 -> [w364 w366]
              tunnel: w357 -> [w363 _]
              tunnel: w354 -> [w362 _]
              frame True {
                n175 = invoke class="VI" method="FP.Open"(reference=w363, error in=w364, "State"=w362) -> (error out=w365:errorcluster)  [unwired: 2 in, 4 out]
              }
              frame False {
              }
            }
          }
          frame "Minimize", "Minimized" {
            w367 = T3."Minimized" ("State")
            n176 = property class="VI"(reference=w373, error in=w372) -> (reference out=w370:refnum<vi>, error out=w371:errorcluster, "FP.State"=w369:T3)
            n177 = Not Equal?(x=w369, y=w367) -> (x != y?=w368:bool)
            n178 = case shown="True" w368 {
              tunnel: [w378 w379] -> w374
              tunnel: w371 -> [w377 w379]
              tunnel: w370 -> [w376 _]
              tunnel: w367 -> [w375 _]
              frame True {
                n179 = invoke class="VI" method="FP.Open"(reference=w376, error in=w377, "State"=w375) -> (error out=w378:errorcluster)  [unwired: 2 in, 4 out]
              }
              frame False {
              }
            }
          }
          frame "Maximize", "Maximized" {
            w380 = T3."Maximized" ("State")
            n180 = property class="VI"(reference=w386, error in=w385) -> (reference out=w383:refnum<vi>, error out=w384:errorcluster, "FP.State"=w382:T3)
            n181 = Not Equal?(x=w382, y=w380) -> (x != y?=w381:bool)
            n182 = case shown="True" w381 {
              tunnel: [w391 w392] -> w387
              tunnel: w384 -> [w390 w392]
              tunnel: w383 -> [w389 _]
              tunnel: w380 -> [w388 _]
              frame True {
                n183 = invoke class="VI" method="FP.Open"(reference=w389, error in=w390, "State"=w388) -> (error out=w391:errorcluster)  [unwired: 2 in, 4 out]
              }
              frame False {
              }
            }
          }
        }
        n184 = call <vilib>:"Add State(s) to Queue__jki_lib_state_machine.vi"("State(s) in (\"\")"=w327) -> ("States Out"=w326:string)  [unwired: 14 in]
      }
      frame "---------- Macro ----------" {
        # "Do not put any code in this frame.\n(It is a separator no-op. You can make a copy of this frame to create a new Macro frame)"
        n185 = call <vilib>:"Add State(s) to Queue__jki_lib_state_machine.vi"("State(s) in (\"\")"=w396) -> ("States Out"=w395:string)  [unwired: 14 in]
      }
      frame "Macro: Initialize" {
        w397 = "Data: Initialize\nInitialize Core Data\nUI: Initialize\nUI: Front Panel State >> Maximize\nCommunication: Open Serial\nCommunication: 读运行标志"  # Data: Initialize Initialize Core Data UI: Initialize UI: Front Panel State >> Maximize Communication: Open Serial Communication: 读运行标志
        # "Initialization Macro\n(This is called once, when the VI starts)"
        n186 = call <vilib>:"Add State(s) to Queue__jki_lib_state_machine.vi"("State(s) in Front (\"\")"=w397, "State(s) in (\"\")"=w401) -> ("States Out"=w400:string)  [unwired: 13 in]
      }
      frame "Macro: Exit" {
        # "Exit Macro\n(This is called once, when the VI exits)"
        n187 = Unbundle By Name(w408) -> ("Core.Close Panel on Exit?"=w407:bool)
        n188 = disable-structure shown="禁用" {
          frame Disabled {
            n189 = call "mes~设备状态采集.vi"("设备状态"="SHUTDOWN") -> ()  [unwired: 8 in, 3 out]
          }
          frame Enabled {
          }
        }
        n190 = Select(t="UI: Front Panel State >> Close", s=w407, f="") -> (s? t:f=w404:string)
        n191 = call <vilib>:"Add State(s) to Queue__jki_lib_state_machine.vi"("State(s) in (\"\")"=w404, "State(s) at Back (\"\")"="Data: Cleanup\nExit") -> ("States Out"=w402:string)  [unwired: 13 in]
        n192 = call <vilib>:"Add State(s) to Queue__jki_lib_state_machine.vi"("State(s) in Front (\"\")"=w402, "State(s) in (\"\")"=w411) -> ("States Out"=w410:string)  [unwired: 13 in]
      }
      frame "---------- Communication ----------" {
        # "Template Separator\n(You can make a copy of, or modify, this frame)"
        n193 = call <vilib>:"Add State(s) to Queue__jki_lib_state_machine.vi"("State(s) in (\"\")"=w416) -> ("States Out"=w415:string)  [unwired: 14 in]
      }
      frame "Communication: Open Serial" {
        # "Your code here.\n(You can make a copy of, or modify, this frame)"
        n194 = call "读取配置文件.vi"("error in"=w429, "配置"="串口号") -> ("error out"=w428:errorcluster, "路径"=w427:string)  [unwired: 8 in]
        n195 = call "开机连接.vi"("error in"=w428, "波特率"=u32 19200, "串口号"=w427) -> ("error out"=w421:errorcluster, "连接成功"=w423:bool, "serial master instance"=w425:refnum<class "Modbus Master.lvclass">)  [unwired: 6 in]
        n196 = disable-structure shown="Enabled" {
          disable-tunnel: [w440 _] -> w422
          disable-tunnel: w421 -> [w439 _]
          disable-tunnel: "温湿度" ("配置") -> [w438 _]
          disable-tunnel: [w434 _] -> w418
          disable-tunnel: [w433 TRUE ("连接成功")] -> w417
          frame Disabled {
            n197 = call "读取配置文件.vi"("error in"=w439, "配置"=w438) -> ("error out"=w437:errorcluster, "路径"=w436:string)  [unwired: 8 in]
            n198 = disable-structure shown="Enabled" {
              disable-tunnel: [u32 9600 ("波特率") u32 4800 ("波特率")] -> w435
              frame Disabled {
                # "箱体"
              }
              frame Enabled {
                # "液冷"
              }
            }
            n199 = call "开机连接.vi"("error in"=w437, "波特率"=w435, "串口号"=w436) -> ("error out"=w440:errorcluster, "连接成功"=w433:bool, "serial master instance"=w434:refnum<class "Modbus Master.lvclass">)  [unwired: 6 in]
          }
          frame Enabled {
          }
        }
        n200 = Bundle By Name(cluster=w426, "serial master instance"=w425, "连接成功"=w423, "温度instance"=w418) -> (w424:T7)
        n201 = case shown="True" w417 {
          frame False {
            n202 = One Button Dialog(message="温度串口连接失败。" ("消息")) -> ()  [unwired: 1 in, 1 out]
          }
          frame True {
          }
        }
        n203 = call <vilib>:"Add State(s) to Queue__jki_lib_state_machine.vi"("State(s) in (\"\")"=w432) -> ("States Out"=w431:string)  [unwired: 14 in]
      }
      frame "Communication: 设备启动" {
        # "Your code here.\n(You can make a copy of, or modify, this frame)"
        n204 = Unbundle By Name(w452) -> ("serial master instance"=w453:refnum<class "Modbus Master.lvclass">, "连接成功"=w454:bool, "用户登录"=w447:bool, "进站OK"=w446:bool)
        n205 = And(x=w447, y=w446) -> (x .and. y?=w448:bool)
        n206 = case shown="False" w448 {
          tunnel: w456 -> [w461 w473]
          tunnel: [w461 w472] -> w455
          tunnel: w454 -> [w462 w471]
          tunnel: w453 -> [_ w470]
          tunnel: [w462 w469] -> w451
          tunnel: FALSE ("正在运行") -> [w463 w468]
          tunnel: [w463 w467] -> w445
          tunnel: w447 -> [w460 _]
          tunnel: w446 -> [w459 _]
          frame False {
            n207 = case shown="True" w460 {
              tunnel: w459 -> [_ w465]
              frame False {
                n208 = One Button Dialog(message="用户未登录。" ("消息")) -> ()  [unwired: 1 in, 1 out]
              }
              frame True {
                n209 = case shown="False" w465 {
                  frame False {
                    n210 = One Button Dialog(message="产品未进站。" ("消息")) -> ()  [unwired: 1 in, 1 out]
                  }
                  frame True {
                  }
                }
              }
            }
          }
          frame True {
            n211 = case shown="False" w468 {
              selector: w468 -> [_ w493]
              tunnel: w473 -> [w479 w494]
              tunnel: [w478 w494] -> w472
              tunnel: w471 -> [w477 w495]
              tunnel: w470 -> [w476 _]
              tunnel: [w475 w495] -> w469
              tunnel: [w474 w493] -> w467
              frame False {
                n212 = case shown="True" w477 {
                  tunnel: w479 -> [w480 w485]
                  tunnel: [w480 w484] -> w478
                  tunnel: w476 -> [_ w483]
                  tunnel: [_ w482] -> w475
                  tunnel: [_ TRUE] -> w474
                  frame False {
                  }
                  frame True {
                    n213 = stacked-sequence {
                      tunnel: w485 -> [_ w491 _]
                      tunnel: [_ w490 _] -> w484
                      tunnel: w483 -> [_ w489 _]
                      tunnel: [_ w488 _] -> w482
                      frame #0 {
                        n214 = local write "阻断通讯"(TRUE ("阻断通讯")) -> ()
                      }
                      frame #1 {
                        w487 = cluster{"地址":u16, "布尔":bool, "名称":string}[] [{"地址"=50, "布尔"=TRUE, "名称"="启动"}, {"地址"=51, "布尔"=FALSE, "名称"="停止"}]  # A写入线圈信息组
                        n215 = call "写入单个线圈.vi"("error in"=w491, "写入线圈信息组"=w487, "MB_实体"=w489) -> ("输出簇"=w490:errorcluster, "连接成功"=w488:bool)  [unwired: 7 in]
                      }
                      frame #2 {
                        n216 = local write "阻断通讯"(FALSE ("阻断通讯")) -> ()
                      }
                    }
                  }
                }
              }
              frame True {
              }
            }
          }
        }
        n217 = Bundle By Name(cluster=w452, "正在运行"=w445, "连接成功"=w451) -> (w450:T7)
        n218 = call <vilib>:"Add State(s) to Queue__jki_lib_state_machine.vi"("State(s) in (\"\")"=w458) -> ("States Out"=w457:string)  [unwired: 14 in]
      }
      frame "Communication: 设备停止" {
        # "Your code here.\n(You can make a copy of, or modify, this frame)"
        n219 = Unbundle By Name(w501) -> ("serial master instance"=w502:refnum<class "Modbus Master.lvclass">, "连接成功"=w503:bool, "用户登录"=w497:bool)
        n220 = case shown="True" w497 {
          tunnel: w505 -> [w510 w518]
          tunnel: [w510 w517] -> w504
          tunnel: w503 -> [w508 w516]
          tunnel: w502 -> [_ w515]
          tunnel: [w508 w514] -> w500
          tunnel: TRUE ("正在运行") -> [w509 w513]
          tunnel: [w509 w512] -> w498
          frame False {
            n221 = One Button Dialog(message="用户未登录" ("消息")) -> ()  [unwired: 1 in, 1 out]
          }
          frame True {
            n222 = case shown="True" w513 {
              selector: w513 -> [w519 _]
              tunnel: w518 -> [w520 w527]
              tunnel: [w520 w526] -> w517
              tunnel: w516 -> [w521 w525]
              tunnel: w515 -> [_ w524]
              tunnel: [w521 w523] -> w514
              tunnel: [w519 w522] -> w512
              frame False {
              }
              frame True {
                n223 = case shown="True" w525 {
                  tunnel: w527 -> [w529 w534]
                  tunnel: [w529 w533] -> w526
                  tunnel: w524 -> [_ w532]
                  tunnel: [_ w531] -> w523
                  tunnel: [FALSE FALSE] -> w522
                  frame False {
                  }
                  frame True {
                    n224 = stacked-sequence {
                      tunnel: w534 -> [_ w540 _]
                      tunnel: [_ w539 _] -> w533
                      tunnel: w532 -> [_ w538 _]
                      tunnel: [_ w537 _] -> w531
                      frame #0 {
                        n225 = local write "阻断通讯"(TRUE ("阻断通讯")) -> ()
                      }
                      frame #1 {
                        w536 = cluster{"地址":u16, "布尔":bool, "名称":string}[] [{"地址"=50, "布尔"=FALSE, "名称"="启动"}, {"地址"=51, "布尔"=TRUE, "名称"="停止"}]  # A写入线圈信息组
                        n226 = call "写入单个线圈.vi"("error in"=w540, "写入线圈信息组"=w536, "MB_实体"=w538) -> ("输出簇"=w539:errorcluster, "连接成功"=w537:bool)  [unwired: 7 in]
                      }
                      frame #2 {
                        n227 = local write "阻断通讯"(FALSE ("阻断通讯")) -> ()
                      }
                    }
                  }
                }
              }
            }
          }
        }
        n228 = Bundle By Name(cluster=w501, "正在运行"=w498, "连接成功"=w500) -> (w499:T7)
        n229 = call <vilib>:"Add State(s) to Queue__jki_lib_state_machine.vi"("State(s) in (\"\")"=w507) -> ("States Out"=w506:string)  [unwired: 14 in]
      }
      frame "Communication: 读运行标志" {
        n230 = Unbundle By Name(w543) -> ("serial master instance"=w542:refnum<class "Modbus Master.lvclass">)
        n231 = stacked-sequence {
          tunnel: w548 -> [_ w557 _]
          tunnel: [_ w556 _] -> w547
          tunnel: [_ w555 _] -> w546
          tunnel: [_ w554 _] -> w545
          tunnel: w542 -> [_ w552 _]
          frame #0 {
            n232 = local write "阻断通讯"(TRUE ("阻断通讯")) -> ()
          }
          frame #1 {
            w553 = T9 [{"地址"=507, "数量"=1, "名称"="1测试结束标志", "线圈组"=[]}]  # A读多组线圈信息组
            n233 = call "读线圈组.vi"("error in"=w557, "读多组线圈__输入"=w553, "MB_实体"=w552) -> ("输出簇"=w556:errorcluster, "正在运行"=w554:bool, "连接成功"=w555:bool)  [unwired: 6 in]
          }
          frame #2 {
            n234 = local write "阻断通讯"(FALSE ("阻断通讯")) -> ()
          }
        }
        n235 = Bundle By Name(cluster=w543, "连接成功"=w546, "正在运行"=w545) -> (w544:T7)
        n236 = call <vilib>:"Add State(s) to Queue__jki_lib_state_machine.vi"("State(s) in (\"\")"=w550) -> ("States Out"=w549:string)  [unwired: 14 in]
      }
      frame "---------- 设备状态采集 ----------" {
        # "Do not put any code in this frame.\n(it is a separator no-op)"
        n237 = call <vilib>:"Add State(s) to Queue__jki_lib_state_machine.vi"("State(s) in (\"\")"=w562) -> ("States Out"=w561:string)  [unwired: 14 in]
      }
      frame "通讯参数设置" {
        n238 = stacked-sequence {
          tunnel: w564 -> [_ w572 _]
          tunnel: [_ w569 _] -> w563
          frame #0 {
            n239 = local write "阻断通讯"(TRUE ("阻断通讯")) -> ()
          }
          frame #1 {
            n240 = call "通讯参数设置.vi"() -> ("A设备簇"=w573:T8)  [unwired: 5 in]
            n241 = Unbundle By Name(w573) -> ("MB_实体"=w571:refnum<class "Modbus Master.lvclass">, "连接成功"=w570:bool)
            n242 = Bundle By Name(cluster=w572, "serial master instance"=w571, "连接成功"=w570) -> (w569:T7)
          }
          frame #2 {
            n243 = local write "阻断通讯"(FALSE ("阻断通讯")) -> ()
          }
        }
        n244 = call <vilib>:"Add State(s) to Queue__jki_lib_state_machine.vi"("State(s) in (\"\")"=w567) -> ("States Out"=w566:string)  [unwired: 14 in]
      }
    }
  }
